vi "Create Sensor Table.vi"(8 "error in (no error)":errorcluster, 10 "SensorID":i32, 11 "Sensor CoreData":T1[](array[typedef])) -> (0 "error out":errorcluster, 3 "Session Table":string[][](array[string]))   [LabVIEW 2026, in "Analysis.lvlib"]
uses:
  Analysis.lvlib
  controls/Messaging Payloads/Sensor CoreData Cluster.ctl
  controls/UI/Units Enum.ctl
  controls/UI/Signal Enum.ctl
  Settings/Settings.lvlib
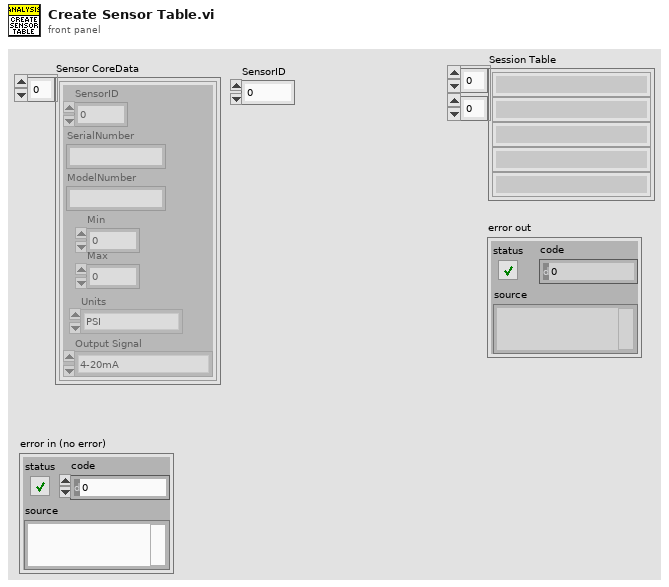
[diagram p1: front panel]
types:
  T1 = typedef "Settings.lvlib/Sensor CoreData Cluster.ctl" = cluster{"SensorID":i32, "SerialNumber":string, "ModelNumber":string, "Min":dbl, "Max":dbl, "Units":T2, "Output Signal":T3}
  T2 = typedef "Units Enum.ctl" = enum16{"PSI", "Deg C", "kPa", "GPM"}
  T3 = typedef "Signal Enum.ctl" = enum16{"4-20mA", "0-10V", "Thermocouple Type K"}
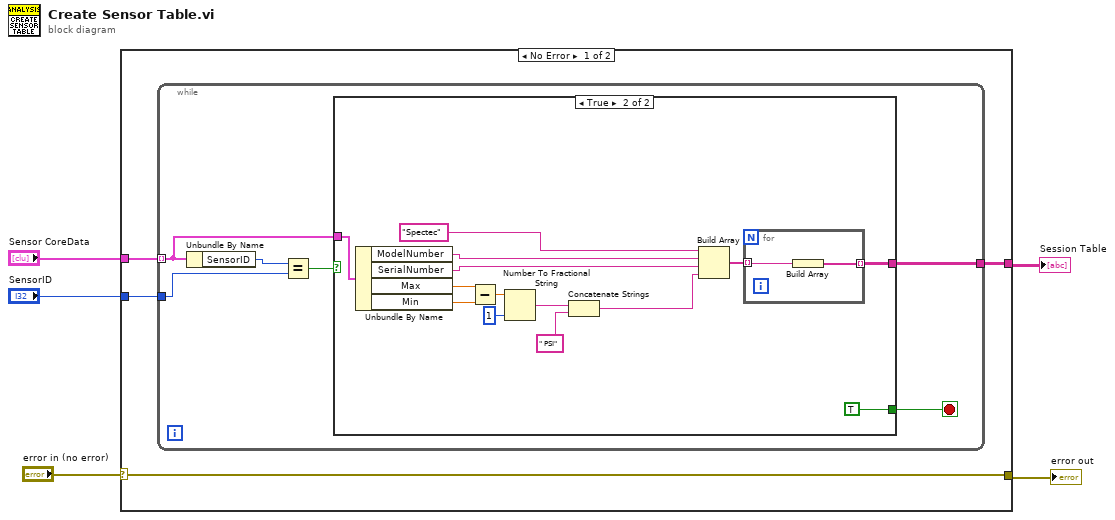
[diagram p0: block diagram]
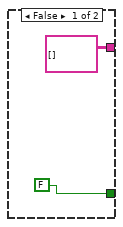
[diagram p2: hidden frame]
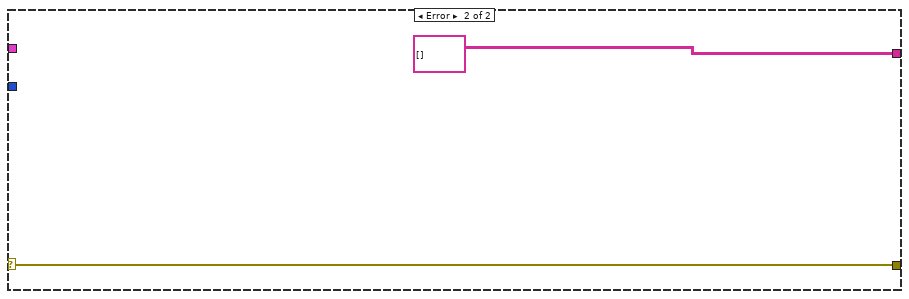
[diagram p3: hidden frame]
diagram:
  n1 = case shown="No Error" "error in (no error)" {
    selector: "error in (no error)" -> [w9 w35]
    tunnel: [w9 w35] -> w4
    tunnel: [w8 string[][] []] -> w3
    tunnel: "Sensor CoreData" -> [w7 _]
    tunnel: "SensorID" -> [w6 _]
    frame No Error {
      n2 = while {
        tunnel: [w15] -> w8
        tunnel: w7 -> [w11] mode=indexing
        tunnel: w6 -> [w13]
        stop <- w10 stop-if-true
        n3 = Unbundle By Name(w11) -> ("SensorID"=w14:i32)
        n4 = Equal?(x=w14, y=w13) -> (x = y?=w12:bool)
        n5 = case shown="True" w12 {
          tunnel: [string[][] [] w29] -> w15
          tunnel: w11 -> [_ w28]
          tunnel: [FALSE TRUE] -> w10
          frame False {
          }
          frame True {
            n6 = Unbundle By Name(w28) -> ("ModelNumber"=w27:string, "SerialNumber"=w26:string, "Max"=w25:dbl, "Min"=w24:dbl)
            n7 = Subtract(x=w25, y=w24) -> (x-y=w23:dbl)
            n8 = Number To Fractional String(number=w23, precision (6)=i16 1) -> (F-format string=w22:string)  [unwired: 2 in]
            n9 = Concatenate Strings(w22, " PSI" ("string")) -> (w20:string)
            n10 = Build Array("Spectec" ("element"), w27, w26, w20) -> (w30:string[])
            n11 = for {
              tunnel: w30 -> [w33] mode=indexing
              tunnel: [w32] -> w29 mode=indexing
              n12 = Build Array(w33) -> (w32:string[])
            }
          }
        }
      }
    }
    frame Error {
    }
  }
  "Session Table" <- w3
  "error out" <- w4
